vi "Initialize Stim Parameters.vi"(4 "Stimulator in":T2={"Log File In"=refnum, "Stimulator In"="", "Stimulator Mode"="", "Log Data"=FALSE, "Doublet/Triplet  Interval"=0.0, "Stim Frequency"=0.0, "N-Factor"=0, "Active Channels"=[], "Low-Frequency Channels"=[], "Stimulator State"=enum."Closed", "Mode Array"=[], "Current Array"=[], "Pulse Duration Array"=[], "VISA Timeout"=50}, 5 "Default Stimulator Parameters":T1) -> (2 "Stimulator out":T2={"Log File In"=refnum, "Stimulator In"="", "Stimulator Mode"="", "Log Data"=FALSE, "Doublet/Triplet  Interval"=0.0, "Stim Frequency"=0.0, "N-Factor"=0, "Active Channels"=[], "Low-Frequency Channels"=[], "Stimulator State"=enum."Closed", "Mode Array"=[], "Current Array"=[], "Pulse Duration Array"=[], "VISA Timeout"=50})   [LabVIEW 2019]
uses:
  Controls/Stimulator Cluster.ctl
  Controls/Stimulator Mode.ctl
  Version 2/Data Type Defs/Pulse Mode (array).ctl
  Controls/Stim Current Array.ctl
  Controls/Pulse Duration Array.ctl
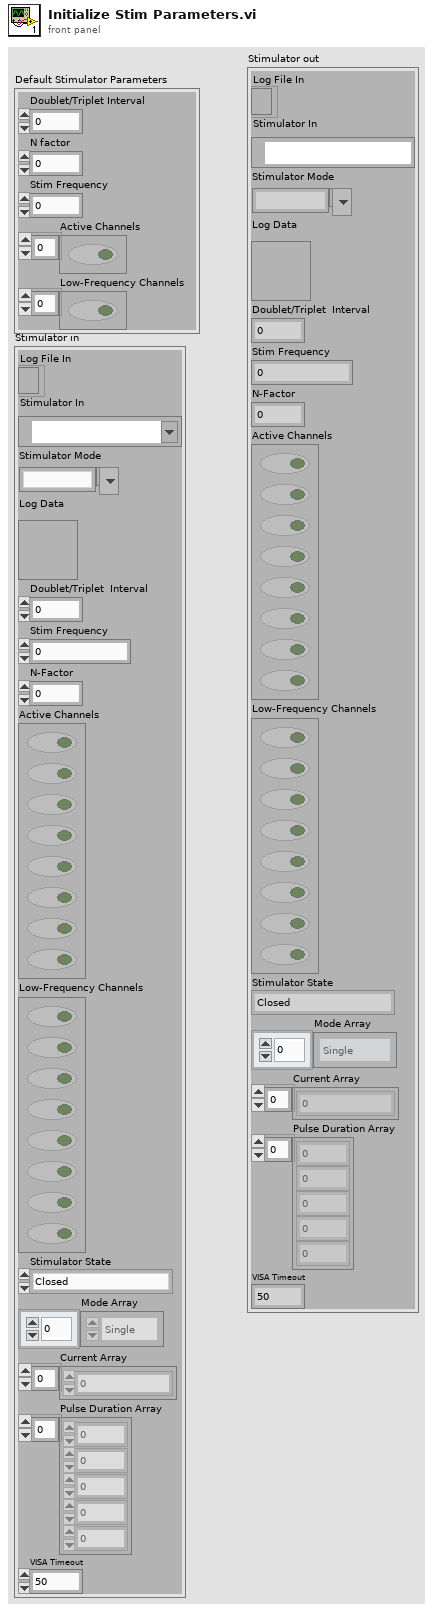
[diagram p1: front panel]
types:
  T1 = cluster{"Doublet/Triplet Interval":dbl, "N factor":u8, "Stim Frequency":dbl, "Active Channels":bool[], "Low-Frequency Channels":bool[]}
  T2 = typedef "Stimulator Cluster.ctl" = cluster{"Log File In":refnum<file>, "Stimulator In":refnum<visa-resource-name>, "Stimulator Mode":T3, "Log Data":bool, "Doublet/Triplet  Interval":dbl, "Stim Frequency":dbl, "N-Factor":u8, "Active Channels":bool[], "Low-Frequency Channels":bool[], "Stimulator State":enum16{"Closed", "Open", "Initialized", "Stimulating"}, "Mode Array":T4, "Current Array":T5, "Pulse Duration Array":T6, "VISA Timeout":u32}
  T3 = typedef "Stimulator Mode.ctl" = string
  T4 = typedef "Pulse Mode (array).ctl" = enum16{"Single", "Doublet", "Triplet"}[]
  T5 = typedef "Stim Current Array.ctl" = u8[]
  T6 = typedef "Pulse Duration Array.ctl" = u32[]
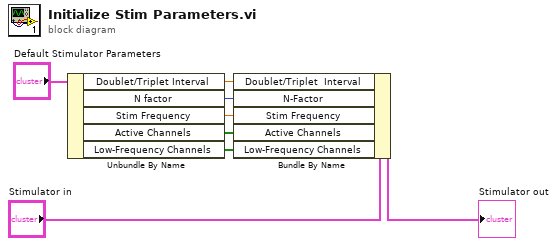
[diagram p0: block diagram]
diagram:
  n1 = Unbundle By Name("Default Stimulator Parameters") -> ("Doublet/Triplet Interval"=w2:dbl, "N factor"=w3:u8, "Stim Frequency"=w4:dbl, "Active Channels"=w5:bool[], "Low-Frequency Channels"=w6:bool[])
  n2 = Bundle By Name(cluster="Stimulator in", "Doublet/Triplet  Interval"=w2, "N-Factor"=w3, "Stim Frequency"=w4, "Active Channels"=w5, "Low-Frequency Channels"=w6) -> (→"Stimulator out":T2)
